vi "MeasurementItems_ClearChannels.vi"(8 "error in (no error)":errorcluster, 10 "#Channel (-1 for all)":i32[](array[numeric]), 11 "OXY_SCPI Reseource In":refnum<visa-resource-name>) -> (0 "error out":errorcluster, 1 "communication_data":T1, 3 "OXY_SCPI Reseource Out":refnum<visa-resource-name>)   [LabVIEW 2018, in "OXYGEN.lvlib"]
doc: "Clear (Set to NONE) given items."
uses:
  OXYGEN.lvlib
  TypeDefs/Cluster_RawCommData.ctl
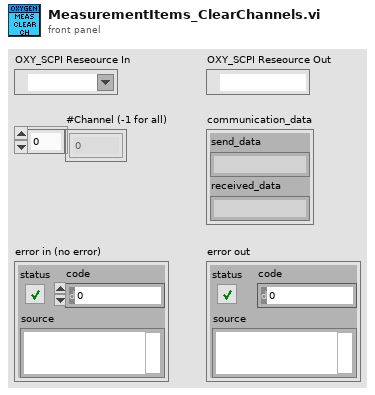
[diagram p1: front panel]
types:
  T1 = typedef "OXYGEN.lvlib/Cluster_RawCommData.ctl" = cluster{"send_data":string, "received_data":string}
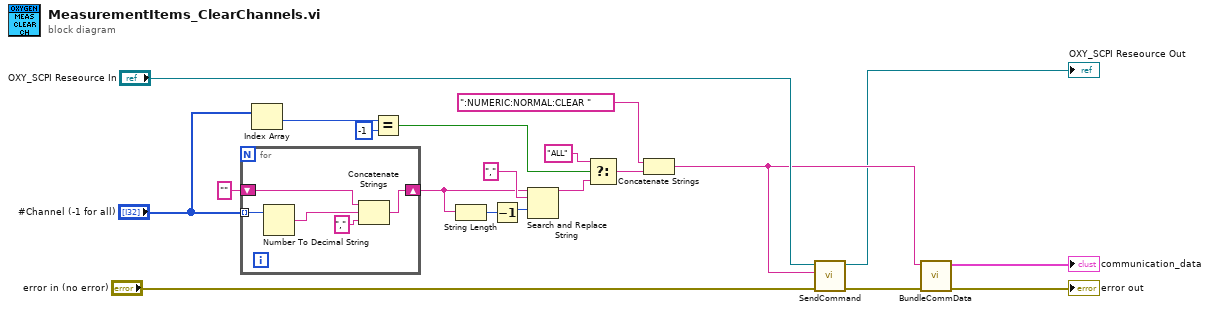
[diagram p0: block diagram]
diagram:
  n1 = for {
    tunnel: "#Channel (-1 for all)" -> [w23] mode=indexing
    shift-right: [w24] -> w11
    shift-left: "" -> [w21]
    n2 = Number To Decimal String(number=w23) -> (decimal integer string=w22:string)  [unwired: 1 in]
    n3 = Concatenate Strings(w21, w22, "," ("string")) -> (w24:string)
  }
  n4 = Index Array(array="#Channel (-1 for all)") -> (element=w16:i32)  [unwired: 1 in]
  n5 = Equal?(x=w16, y=-1) -> (x = y?=w7:bool)
  n6 = String Length(string=w11) -> (length=w10:i32)
  n7 = Decrement(x=w10) -> (x-1=w13:i32)
  n8 = Search and Replace String(input string=w11, search string=",", offset=w13) -> (result string=w8:string)  [unwired: 5 in, 3 out]
  n9 = Select(t="ALL", s=w7, f=w8) -> (s? t:f=w4:string)
  n10 = Concatenate Strings(":NUMERIC:NORMAL:CLEAR " ("t"), w4) -> (w3:string)
  n11 = call "SendCommand.vi"("error in (no error)"="error in (no error)", "String to Send"=w3, "OXY_SCPI Reseource In"="OXY_SCPI Reseource In") -> ("error out"=w2:errorcluster, "OXY_SCPI Reseource Out"=→"OXY_SCPI Reseource Out":refnum<visa-resource-name>)  [unwired: 7 in]
  n12 = call "BundleCommData.vi"("error in (no error)"=w2, "send_data"=w3) -> ("error out"=→"error out":errorcluster, "communication_data"=→"communication_data":T1)  [unwired: 8 in]
